vi "Main.vi"() -> ()   [LabVIEW 2017]
uses:
  <vilib>/addons/database/Connection.llb/Conn ObjectReference.ctl
  <vilib>/addons/database/Connection.llb/DB Tools Open Connec (Path).vi
  <vilib>/addons/database/Connection.llb/Conn Execute.vi
  <vilib>/addons/database/Recordset.llb/Rec Fetch Recordset Data (R).vi
  <vilib>/addons/database/Recordset.llb/Rec Destroy - Connection.vi
  <vilib>/addons/database/NI_Database_API.lvlib
panel:
  out "Current Time":string
  out "Current Date":string
  out "1D Array":string[](array[string])=["01:00 - 01:59", "02:00 - 02:59", "03:00 - 03:59", "04:00 - 04:59", "05:00 - 05:59", "06:00 - 06:59", "07:00 - 07:59", "08:00 - 08:59", "09:00 - 09:59", "10:00 - 10:59", "11:00 - 11:59", "12:00 - 12:59", "13:00 - 13:59", "14:00 - 14:59", "15:00 - 15:59", "16:00 - 16:59", "17:00 - 17:59", "18:00 - 18:59", "19:00 - 19:59", "20:00 - 20:59", "21:00 - 21:59", "22:00 - 22:59", "22:00 - 22:59", "00:00 - 01:59"]
  out "String Indicator 9":string="BREAKDOWN COUNT"
  out "String Indicator":string="PRODUCTION COUNT"
  out "String Indicator 8":string="REJECTION COUNT"
  out "Dlt Cnt":i32
  out "Table 2":string[][][](array[string])
  out "connection reference":T1
  out "String Indicator 1":string="RUNNING..."
  out "BDWn1":dbl
  out "Rej1":dbl
  out "Prod1":dbl
  out "Total Bdwn Time":timestamp format="%<%H:%M:%S>T"
  out "Hourly1":dbl[](array[numeric])
  out "BSWN3":dbl
  out "Rej3":dbl
  out "Prod 3":dbl
  out "Total Bdwn Time3":timestamp format="%<%H:%M:%S>T"
  out "String Indicator 3":string="RUNNING..."
  out "Hourly3":dbl[](array[numeric])
  out "BDWN2":dbl
  out "Rej2":dbl
  out "Prod 2":dbl
  out "Total Bdwn Time2":timestamp format="%<%H:%M:%S>T"
  out "String Indicator 2":string="RUNNING..."
  out "Hourly2":dbl[](array[numeric])
  out "BDWN6":dbl
  out "Rej6":dbl
  out "Prod6":dbl
  out "Total Bdwn Time4":timestamp format="%<%H:%M:%S>T"
  out "String Indicator 6":string="RUNNING..."
  out "Hourly6":dbl[](array[numeric])
  out "BDWN5":dbl
  out "Rej5":dbl
  out "Prod5":dbl
  out "Total Bdwn Time5":timestamp format="%<%H:%M:%S>T"
  out "String Indicator 5":string="RUNNING..."
  out "Hourly5":dbl[](array[numeric])
  out "BDWN4":dbl
  out "Rej4":dbl
  out "Prod4":dbl
  out "Total Bdwn Time6":timestamp format="%<%H:%M:%S>T"
  out "String Indicator4":string="RUNNING..."
  out "Hourly4":dbl[](array[numeric])
  out "Numeric Indicator 4":string=" BREAKDOWN TIME "
  out "Numeric Indicator 3":string="STATUS"
  in  "Cancel Button - Archive":bool
  # "Main Screen"
  # "Station_1"
  # "Station_2"
  # "Station_3"
  # "Station_4"
  # "Station_5"
  # "Station_6"
  # "Designed & Developed By: Infinity Automation Systems Pvt. Ltd."
  # "00.00.53\n00.00.25\n00.00.21\n00.00.15\n11\n7\n2\n8\n1.6\n49\n35\n32\n27"
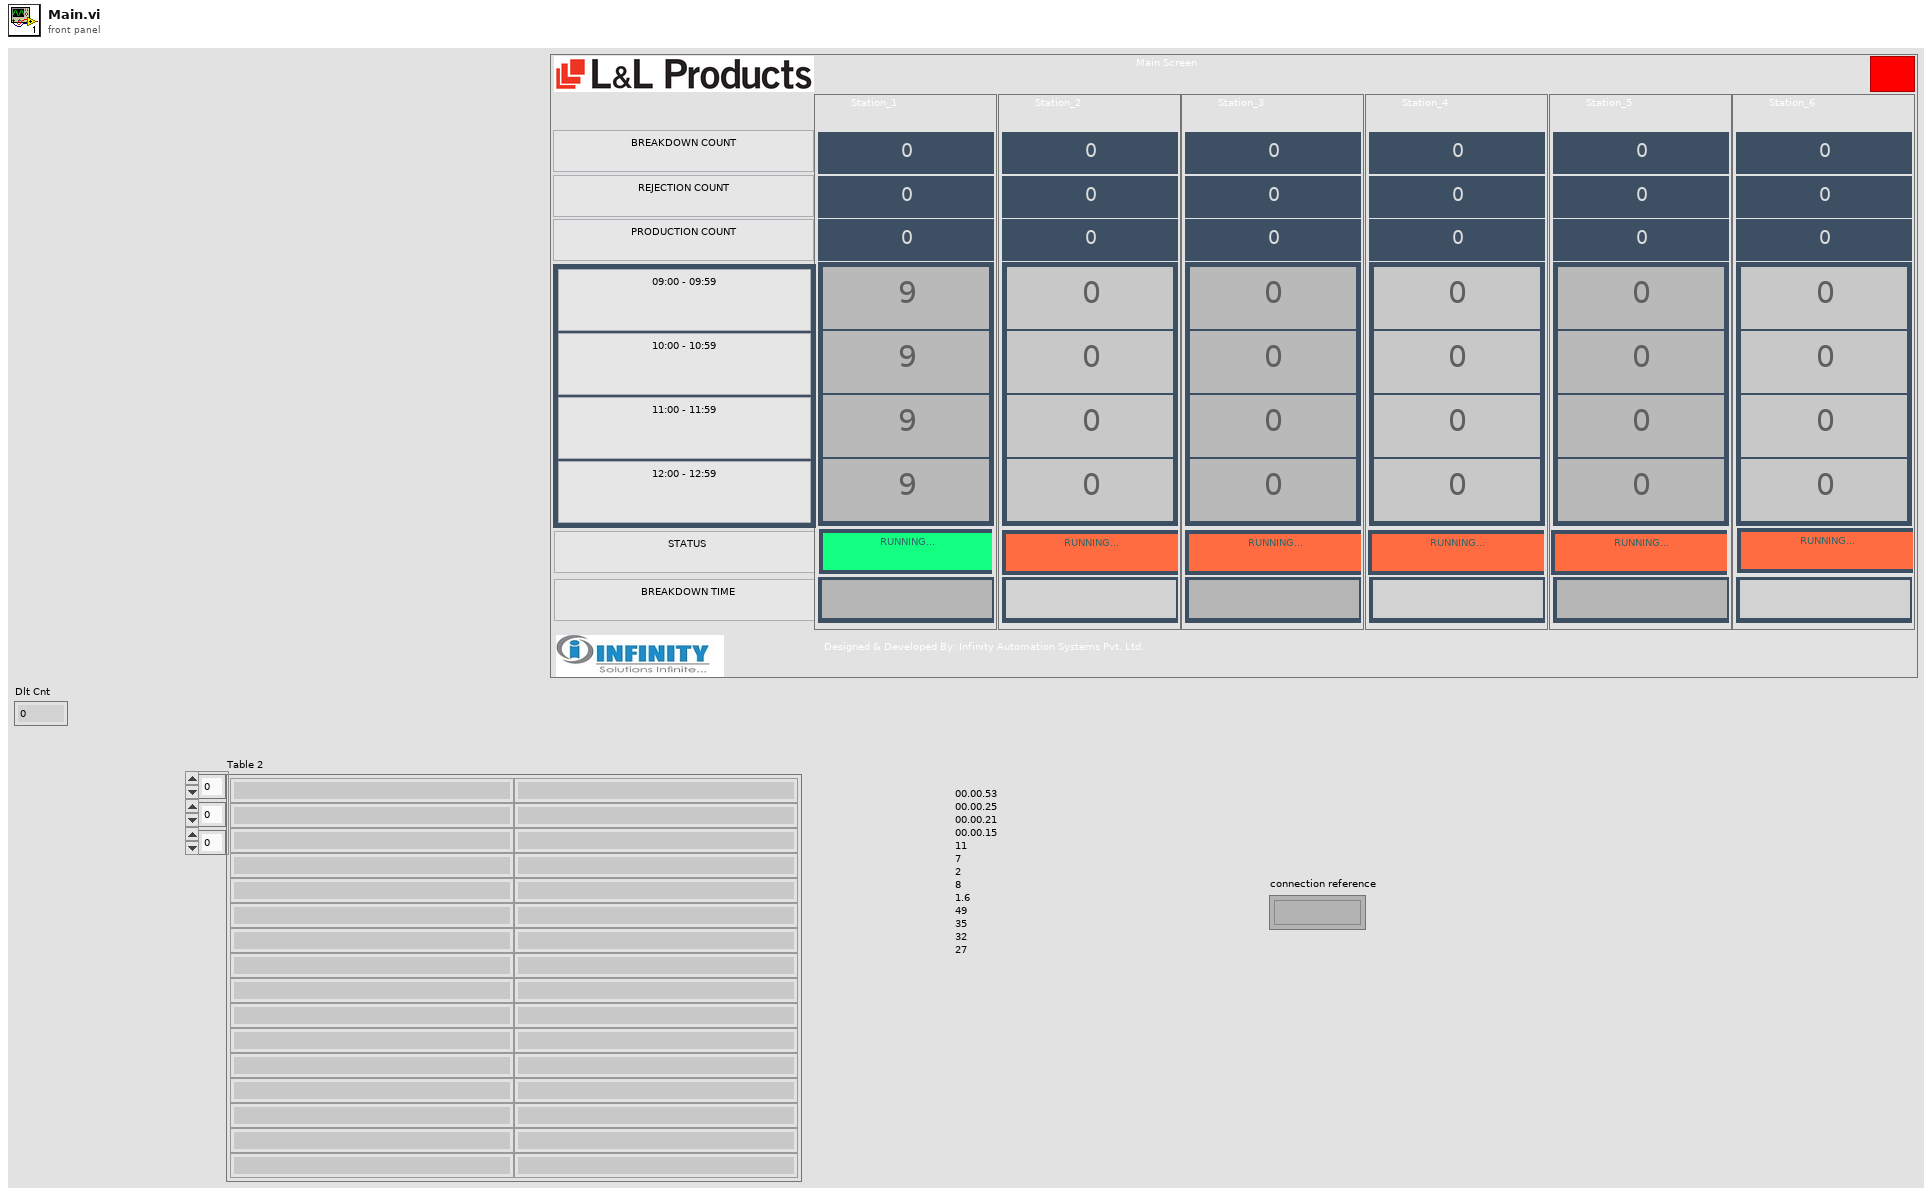
[diagram p1: front panel]
types:
  T1 = typedef "NI_Database_API.lvlib/Conn ObjectReference.ctl" = refnum<k1>
  T2 = typedef "NI_Database_API.lvlib/Rec ObjectReference.ctl" = refnum<k1>
  T3 = enum32{"invalid app kind", "Development System", "Run Time System", "Student Edition", "Embedded LabVIEW", "Evaluation", "Custom"}
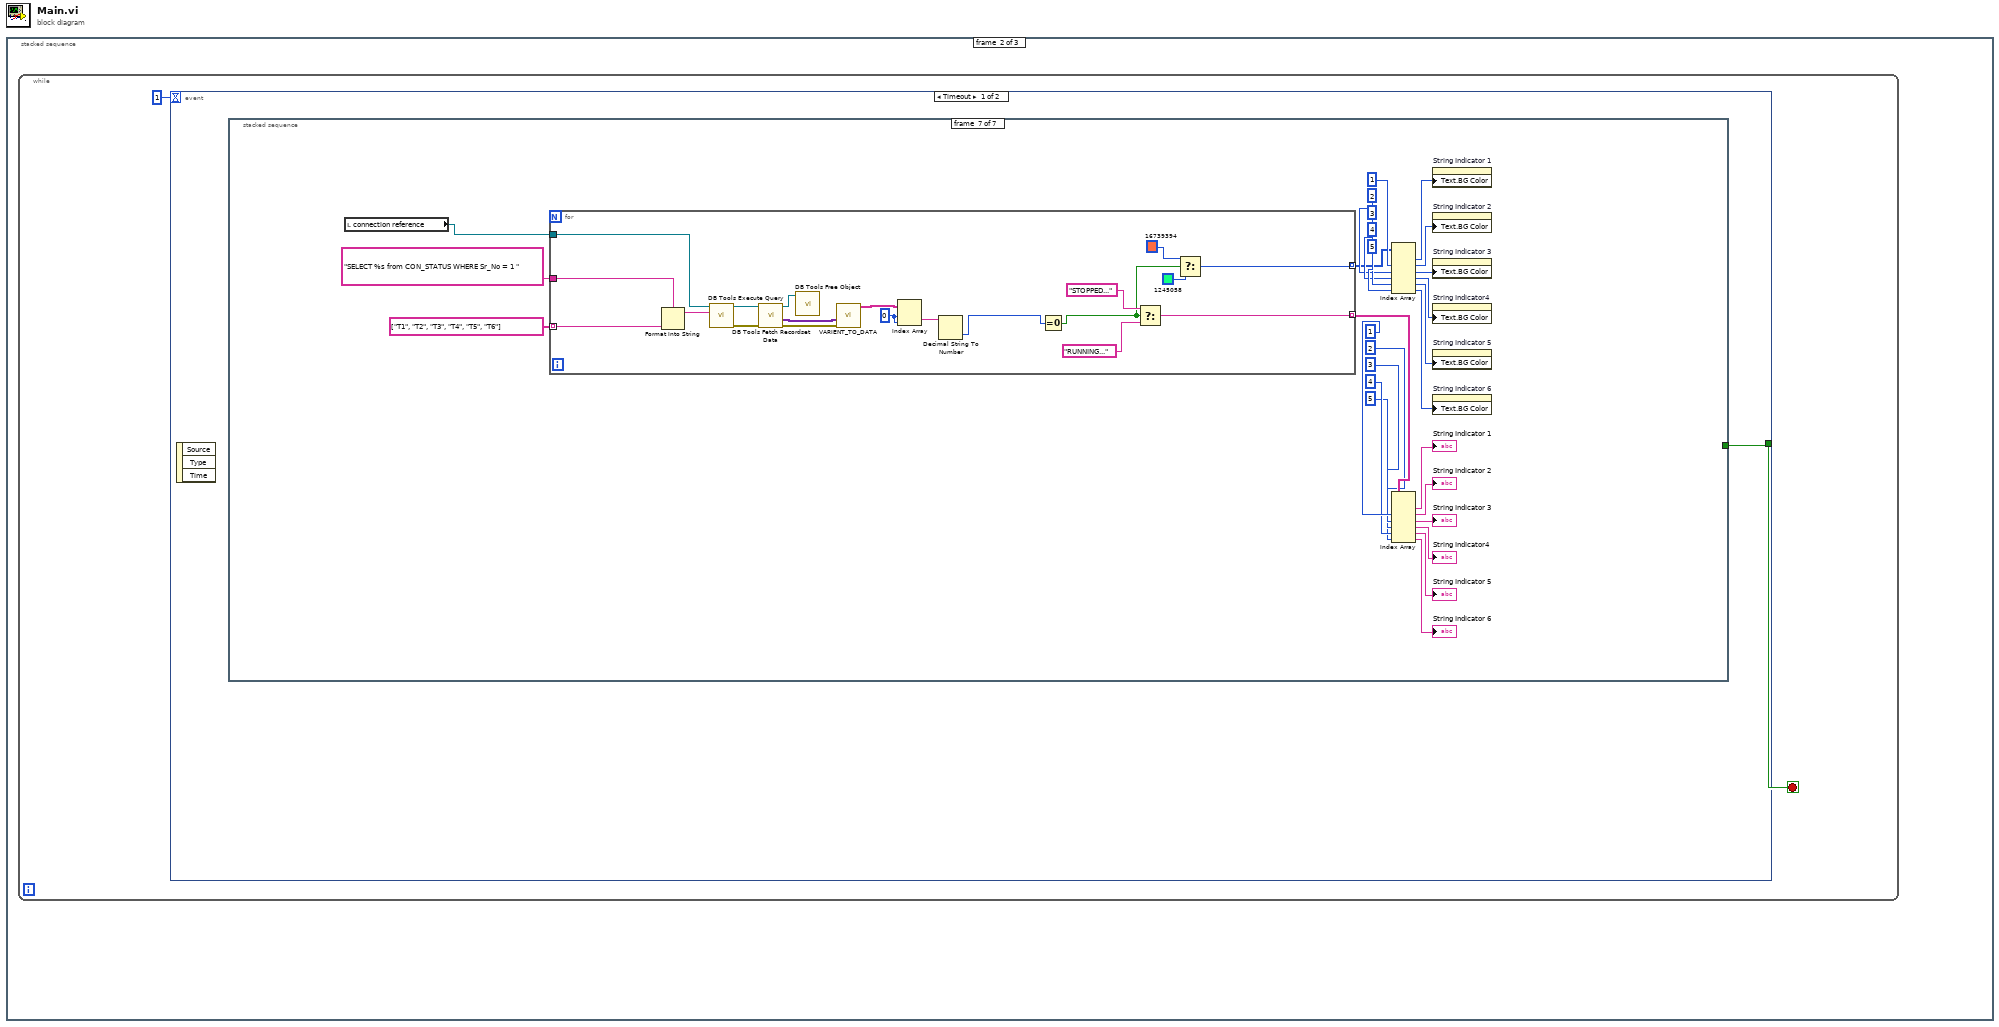
[diagram p0: block diagram]
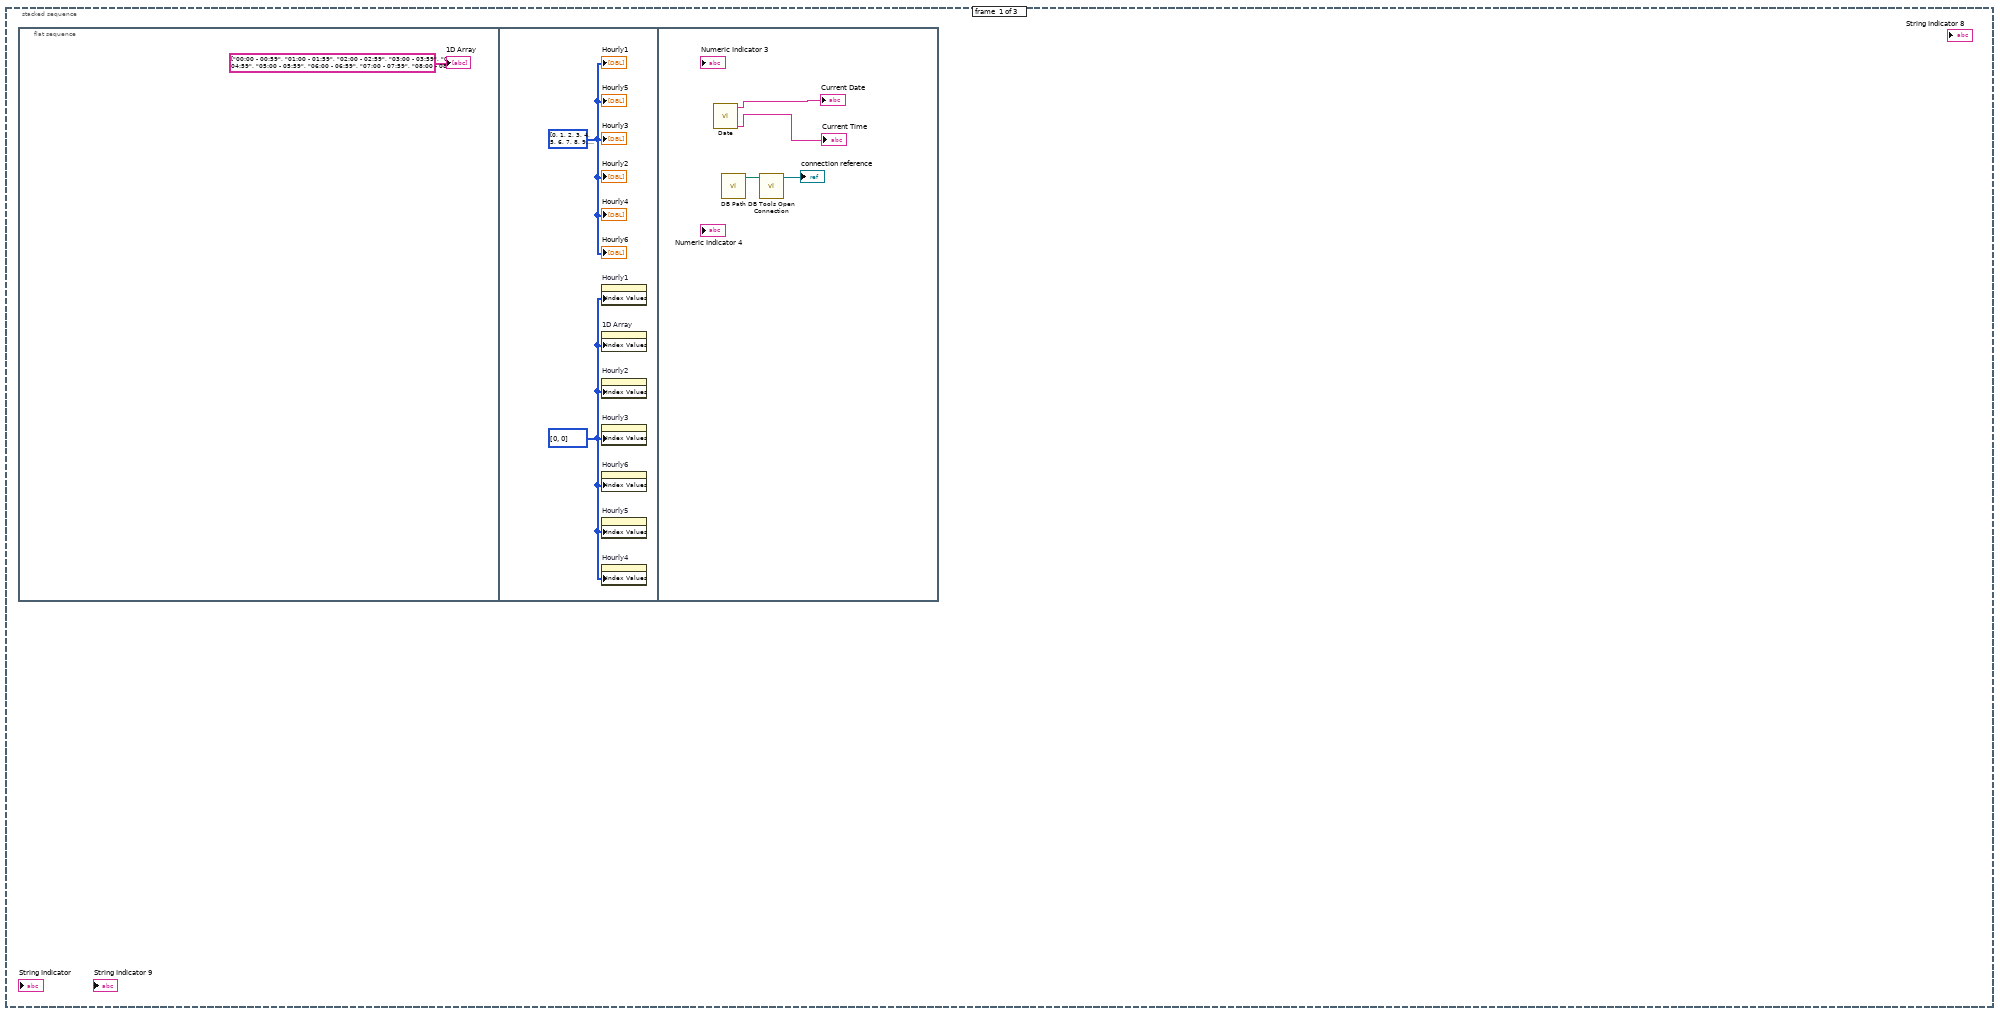
[diagram p2: hidden frame]
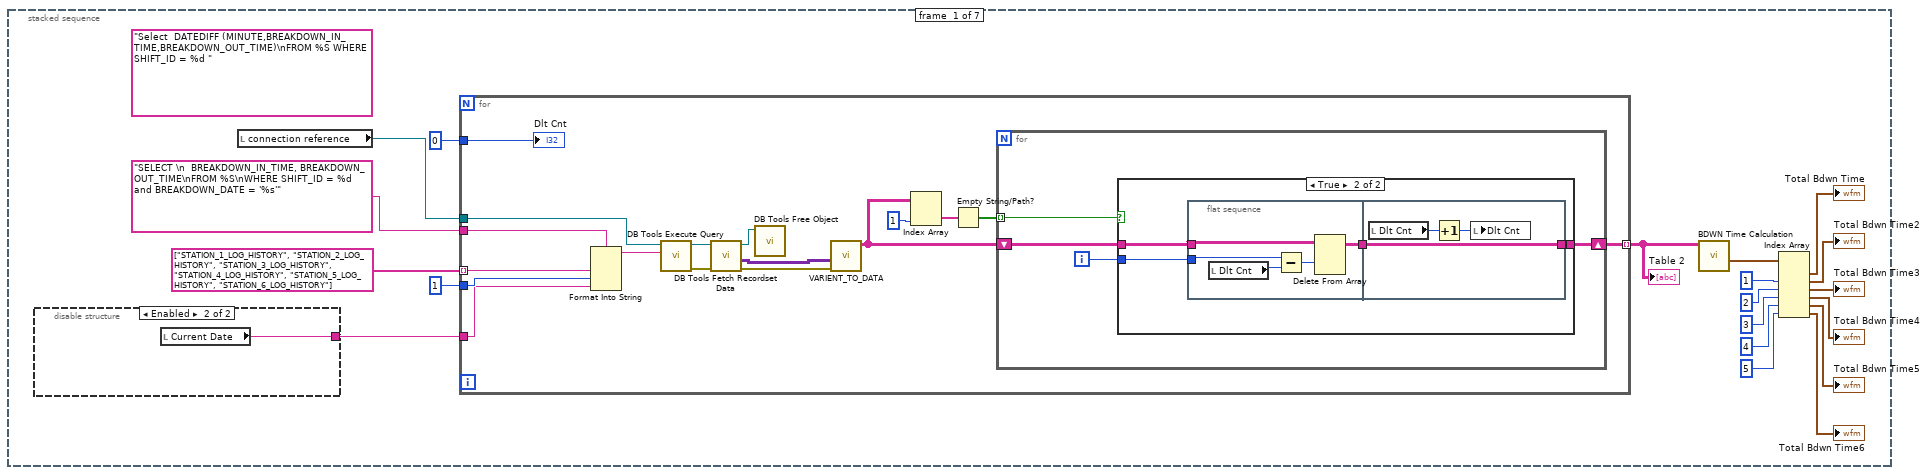
[diagram p3: hidden frame]
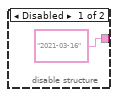
[diagram p4: hidden frame]
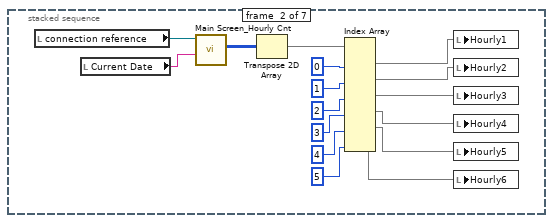
[diagram p6: hidden frame]
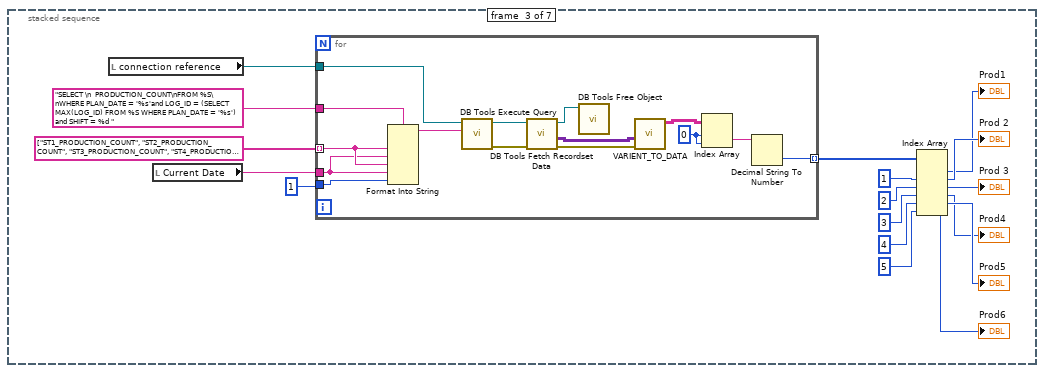
[diagram p7: hidden frame]
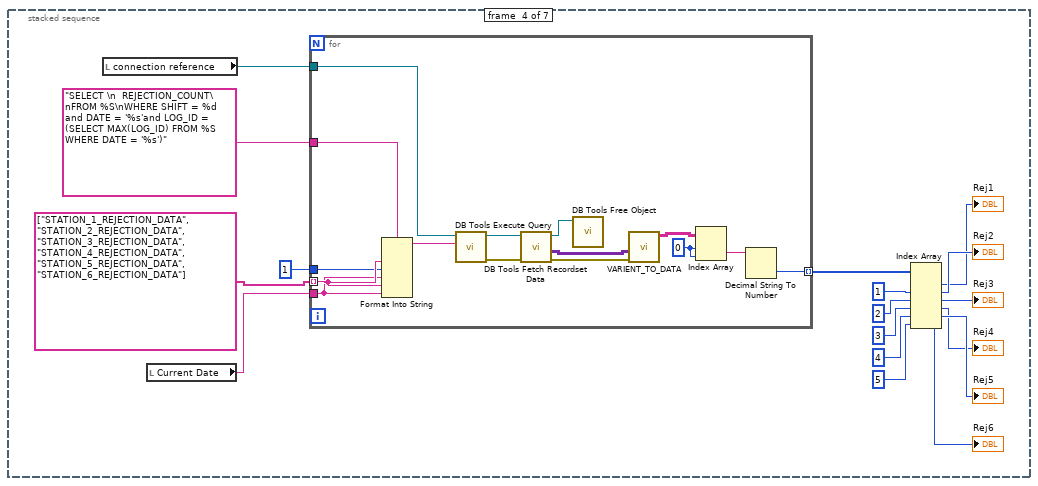
[diagram p8: hidden frame]
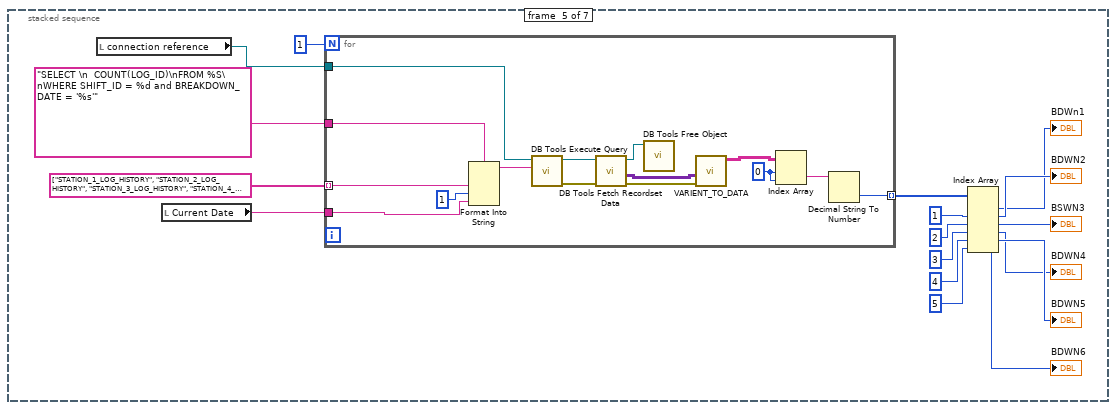
[diagram p9: hidden frame]
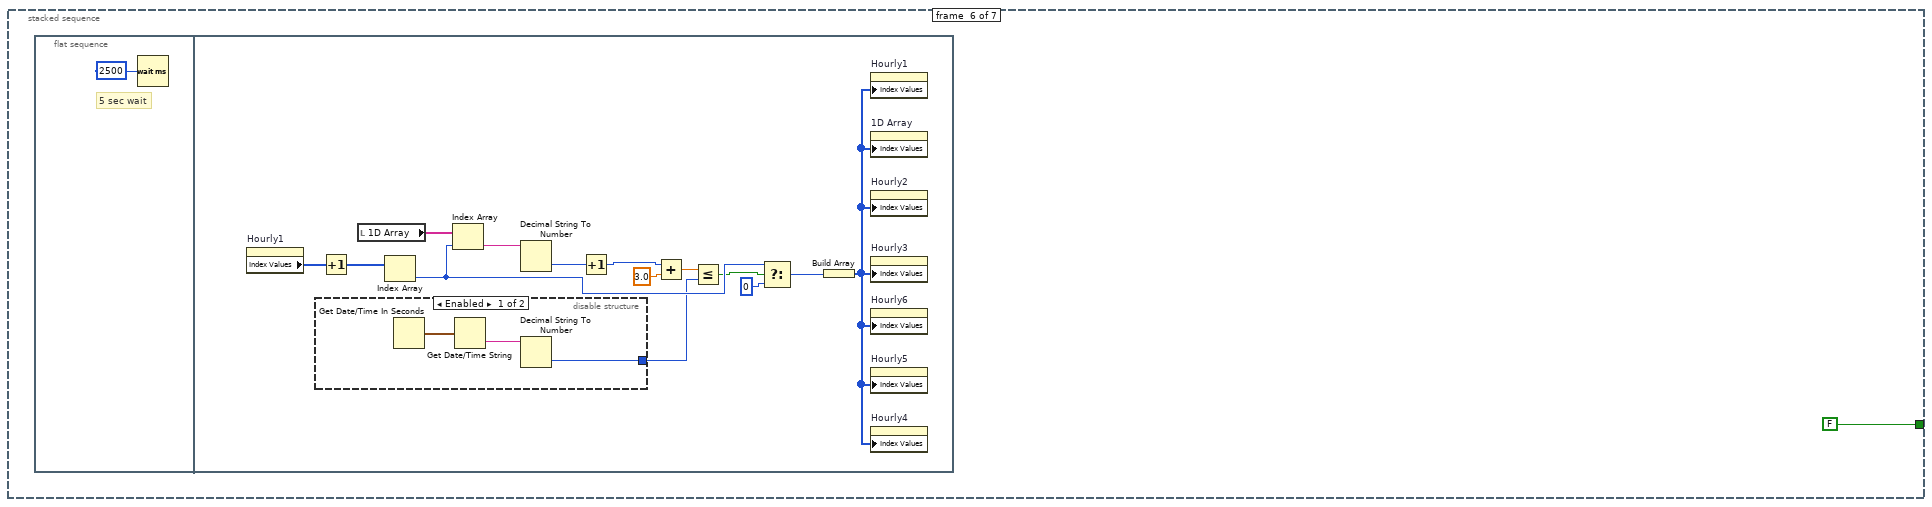
[diagram p10: hidden frame]
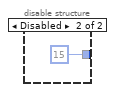
[diagram p11: hidden frame]
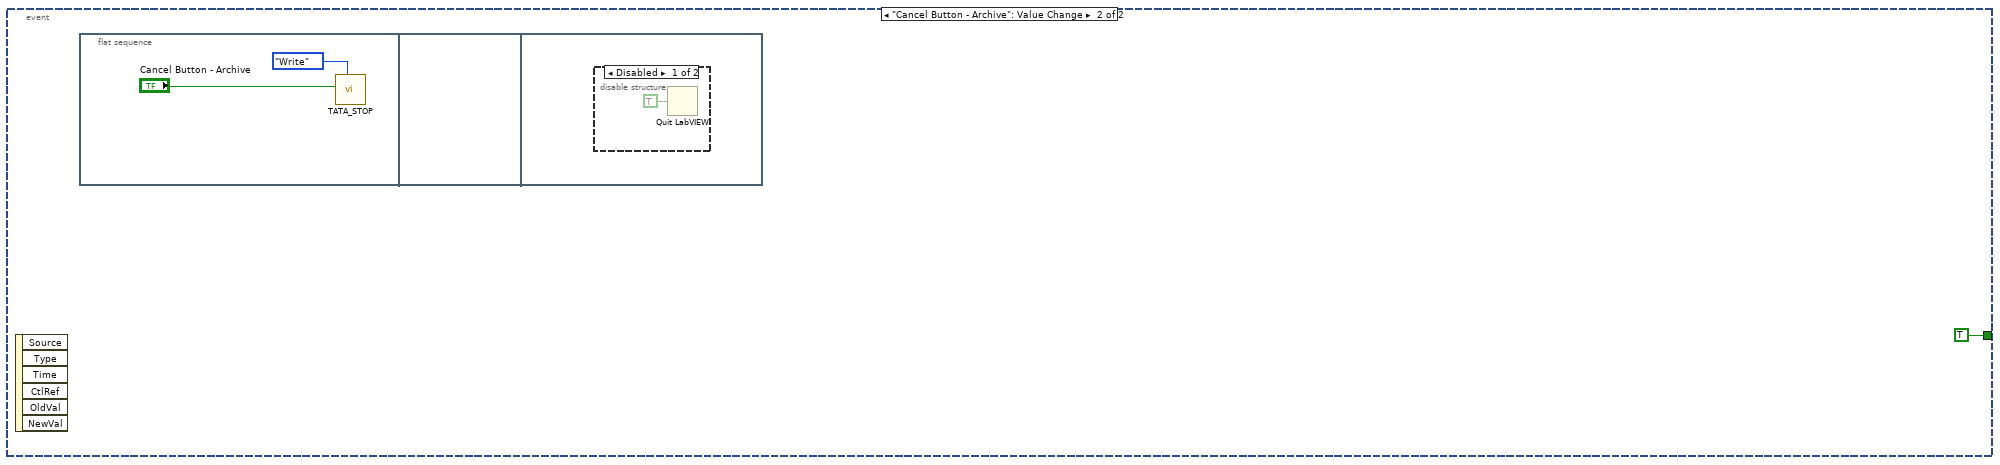
[diagram p12: hidden frame]
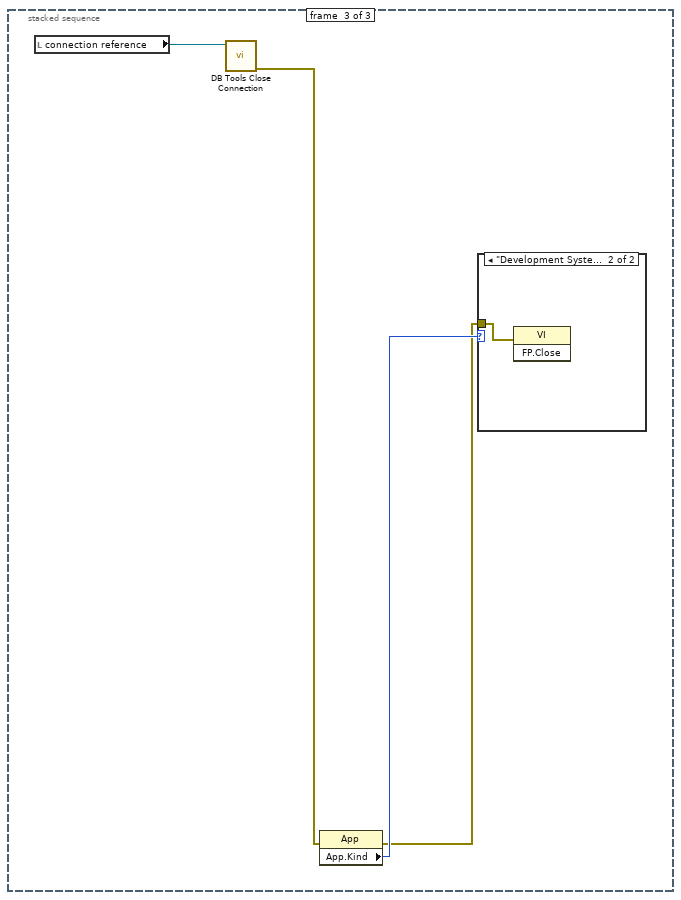
[diagram p14: hidden frame]
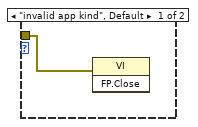
[diagram p15: hidden frame]
diagram:
  n1 = stacked-sequence {
    frame #0 {
      n2 = flat-sequence {
        frame #0 {
          "1D Array" <- string[] ["00:00 - 00:59", "01:00 - 01:59", "02:00 - 02:59", "03:00 - 03:59", "04:00 - 04:59", "05:00 - 05:59", "06:00 - 06:59", "07:00 - 07:59", "08:00 - 08:59", "09:00 - 09:59", "10:00 - 10:59", "11:00 - 11:59", "12:00 - 12:59", "13:00 - 13:59", "14:00 - 14:59", "15:00 - 15:59", "16:00 - 16:59", "17:00 - 17:59", "18:00 - 18:59", "19:00 - 19:59", "20:00 - 20:59", "21:00 - 21:59", "22:00 - 22:59", "23:00 - 23:59"] ("array w/ subset deleted")
        }
        frame #1 {
          w3 = u32[] [0, 1, 2, 3, 4, 5, 6, 7, 8, 9, 10] ("appended array")
          w2 = u32[] [0, 0] ("appended array")
          n3 = property on="Hourly1" class="Arr (strict)"("Index Values"=w2) -> ()  [unwired: 2 in, 2 out]
          n4 = property on="1D Array" class="Arr (strict)"("Index Values"=w2) -> ()  [unwired: 2 in, 2 out]
          n5 = property on="Hourly2" class="Arr (strict)"("Index Values"=w2) -> ()  [unwired: 2 in, 2 out]
          n6 = property on="Hourly3" class="Arr (strict)"("Index Values"=w2) -> ()  [unwired: 2 in, 2 out]
          n7 = property on="Hourly6" class="Arr (strict)"("Index Values"=w2) -> ()  [unwired: 2 in, 2 out]
          n8 = property on="Hourly5" class="Arr (strict)"("Index Values"=w2) -> ()  [unwired: 2 in, 2 out]
          n9 = property on="Hourly4" class="Arr (strict)"("Index Values"=w2) -> ()  [unwired: 2 in, 2 out]
          "Hourly1" <- w3
          "Hourly5" <- w3
          "Hourly3" <- w3
          "Hourly2" <- w3
          "Hourly4" <- w3
          "Hourly6" <- w3
        }
        frame #2 {
          n10 = call "Date.vi"() -> ("Current Time"=→"Current Time":string, "YYYYMMDD Date"=→"Current Date":string)  [unwired: 10 in]
          n11 = call "DB Path.vi"() -> ("DB Path"=w7:path)  [unwired: 10 in, 1 out]
          n12 = call-poly <vilib>:"DB Tools Open Connection.vi"("connection information"=w7) -> ("connection reference"=→"connection reference":T1)  [unwired: 7 in, 1 out]
        }
      }
    }
    frame #1 {
      n13 = while {
        stop <- w9 stop-if-true
        n14 = event shown="[0] Timeout" {
          selector: _ -> [_ _]
          dyn-events: _ -> [_ _]
          timeout: 1 -> [_ _]
          tunnel: [w10 TRUE] -> w9
          event Timeout {
            n15 = event-data() -> ()  [unwired: 1 in, 3 out]
            n16 = stacked-sequence {
              tunnel: [_ _ _ _ _ FALSE _] -> w10
              frame #0 {
                (unwired) "Select  DATEDIFF (MINUTE,BREAKDOWN_IN_TIME,BREAKDOWN_OUT_TIME)\nFROM %S WHERE SHIFT_ID = %d " ("SQL query")
                n17 = disable-structure shown="Enabled" {
                  disable-tunnel: ["2021-03-16" w31] -> w11
                  frame Disabled {
                  }
                  frame Enabled {
                    n18 = local read "Current Date"() -> (w31:string)
                  }
                }
                n19 = local read "connection reference"() -> (w28:T1)
                n20 = for {
                  tunnel: w28 -> [w48]
                  tunnel: "SELECT \n  BREAKDOWN_IN_TIME, BREAKDOWN_OUT_TIME\nFROM %S\nWHERE SHIFT_ID = %d and BREAKDOWN_DATE = '%s'" ("SQL query") -> [w44]
                  tunnel: string[] ["STATION_1_LOG_HISTORY", "STATION_2_LOG_HISTORY", "STATION_3_LOG_HISTORY", "STATION_4_LOG_HISTORY", "STATION_5_LOG_HISTORY", "STATION_6_LOG_HISTORY"] -> [w42] mode=indexing
                  tunnel: 1 ("input 2") -> [w41]
                  tunnel: 0 ("input 2") -> [w34]
                  tunnel: [w33] -> w25 mode=indexing
                  tunnel: w11 -> [w32]
                  n21 = Format Into String(format string=w44, w42, w41, w32) -> (resulting string=w43:string)  [unwired: 2 in, 1 out]
                  n22 = call-poly <vilib>:"DB Tools Execute Query.vi"("SQL query"=w43, "connection reference"=w48) -> ("error out"=w40:errorcluster, "recordset reference"=w47:T2)  [unwired: 6 in]
                  n23 = call-poly <vilib>:"DB Tools Fetch Recordset Data.vi"("error in (no error)"=w40, "recordset reference"=w47) -> ("error out"=w39:errorcluster, "recordset data"=w45:variant[][], "recordset reference out"=w46:T2)  [unwired: 3 in]
                  n24 = call-poly <vilib>:"DB Tools Free Object.vi"("recordset reference"=w46) -> ()  [unwired: 9 in, 2 out]
                  n25 = call "VARIENT_TO_DATA.vi"("data"=w45, "error in (no error)"=w39) -> ("Table"=w35:string[][])  [unwired: 7 in, 1 out]
                  n26 = Index Array(array=w35, index (col)=1 ("disabled index (col)")) -> (element=w37:string[])  [unwired: 1 in]
                  n27 = Empty String/Path?(string/path=w37) -> (empty?=w36:bool[])
                  n28 = for {
                    tunnel: w36 -> [w52] mode=indexing
                    shift-right: [w49] -> w33
                    shift-left: w35 -> [w51]
                    i -> [w50]
                    n29 = case shown="True" w52 {
                      tunnel: w51 -> [w53 w57]
                      tunnel: w50 -> [_ w56]
                      tunnel: [w53 w55] -> w49
                      frame False {
                      }
                      frame True {
                        n30 = flat-sequence {
                          tunnel: w57 -> [w62]
                          tunnel: w56 -> [w60]
                          tunnel: [w61] -> w54
                          tunnel: [w65] -> w55
                          tunnel: w54 -> [w65]
                          frame #0 {
                            n31 = local read "Dlt Cnt"() -> (w59:i32)
                            n32 = Subtract(x=w60, y=w59) -> (x-y=w58:i32)
                            n33 = Delete From Array(array=w62, index (row)=w58) -> (array with subset deleted=w61:string[][])  [unwired: 2 in, 1 out]
                          }
                          frame #1 {
                            n34 = local read "Dlt Cnt"() -> (w63:i32)
                            n35 = Increment(x=w63) -> (x+1=w64:i32)
                            n36 = local write "Dlt Cnt"(w64) -> ()
                          }
                        }
                      }
                    }
                  }
                  "Dlt Cnt" <- w34
                }
                "Table 2" <- w25
                n37 = call "BDWN Time Calculation.vi"("Input Table"=w25) -> ("All BDWN Time"=w24:timestamp[])  [unwired: 8 in, 1 out]
                n38 = Index Array(array=w24, index #2=1 ("index"), index #3=2 ("index"), index #4=3 ("index"), index #5=4 ("index"), index #6=5 ("index")) -> (element #1=→"Total Bdwn Time":timestamp, element #2=→"Total Bdwn Time2":timestamp, element #3=→"Total Bdwn Time3":timestamp, element #4=→"Total Bdwn Time4":timestamp, element #5=→"Total Bdwn Time5":timestamp, element #6=→"Total Bdwn Time6":timestamp)  [unwired: 1 in]
              }
              frame #1 {
                n39 = local read "connection reference"() -> (w73:T1)
                n40 = local read "Current Date"() -> (w66:string)
                n41 = call "Main Screen_Hourly Cnt.vi"("Current Date"=w66, "connection reference 2"=w73) -> ("Station Wise Max"=w74:i32[][])  [unwired: 9 in]
                n42 = Transpose 2D Array(2D array=w74) -> (transposed array=w75:i32[][])
                n43 = Index Array(array=w75, index (col) #1=0 ("disabled index (col)"), index (col) #2=1 ("index (col)"), index (col) #3=2 ("index (col)"), index (col) #4=3 ("index (col)"), index (col) #5=4 ("index (col)"), index (col) #6=5 ("index (col)")) -> (element #1=w76:i32[], element #2=w77:i32[], element #3=w78:i32[], element #4=w79:i32[], element #5=w80:i32[], element #6=w81:i32[])  [unwired: 6 in]
                n44 = local write "Hourly1"(w76) -> ()
                n45 = local write "Hourly2"(w77) -> ()
                n46 = local write "Hourly3"(w78) -> ()
                n47 = local write "Hourly4"(w79) -> ()
                n48 = local write "Hourly5"(w80) -> ()
                n49 = local write "Hourly6"(w81) -> ()
              }
              frame #2 {
                n50 = local read "connection reference"() -> (w98:T1)
                n51 = local read "Current Date"() -> (w82:string)
                n52 = for {
                  tunnel: w98 -> [w113]
                  tunnel: "SELECT \n  PRODUCTION_COUNT\nFROM %S\nWHERE PLAN_DATE = '%s'and LOG_ID = (SELECT MAX(LOG_ID) FROM %S WHERE PLAN_DATE = '%s') and SHIFT = %d " ("SQL query") -> [w109]
                  tunnel: string[] ["ST1_PRODUCTION_COUNT", "ST2_PRODUCTION_COUNT", "ST3_PRODUCTION_COUNT", "ST4_PRODUCTION_COUNT", "ST5_PRODUCTION_COUNT", "ST6_PRODUCTION_COUNT"] -> [w101] mode=indexing
                  tunnel: [w104] -> w91 mode=indexing
                  tunnel: w82 -> [w100]
                  tunnel: 1 ("index") -> [w99]
                  w106 = 0 ("index (row)")
                  n53 = Format Into String(format string=w109, w101, w100, w101, w100, w99) -> (resulting string=w108:string)  [unwired: 2 in, 1 out]
                  n54 = call-poly <vilib>:"DB Tools Execute Query.vi"("SQL query"=w108, "connection reference"=w113) -> ("error out"=w103:errorcluster, "recordset reference"=w112:T2)  [unwired: 6 in]
                  n55 = call-poly <vilib>:"DB Tools Fetch Recordset Data.vi"("error in (no error)"=w103, "recordset reference"=w112) -> ("error out"=w102:errorcluster, "recordset data"=w110:variant[][], "recordset reference out"=w111:T2)  [unwired: 3 in]
                  n56 = call-poly <vilib>:"DB Tools Free Object.vi"("recordset reference"=w111) -> ()  [unwired: 9 in, 2 out]
                  n57 = call "VARIENT_TO_DATA.vi"("data"=w110, "error in (no error)"=w102) -> ("Table"=w107:string[][])  [unwired: 7 in, 1 out]
                  n58 = Index Array(array=w107, index (row)=w106, index (col)=w106) -> (element=w105:string)
                  n59 = Decimal String To Number(string=w105) -> (number=w104:i32)  [unwired: 2 in, 1 out]
                }
                n60 = Index Array(array=w91, index #2=1 ("index"), index #3=2 ("index"), index #4=3 ("index"), index #5=4 ("index"), index #6=5 ("index")) -> (element #1=→"Prod1":i32, element #2=→"Prod 2":i32, element #3=→"Prod 3":i32, element #4=→"Prod4":i32, element #5=→"Prod5":i32, element #6=→"Prod6":i32)  [unwired: 1 in]
              }
              frame #3 {
                n61 = local read "connection reference"() -> (w130:T1)
                n62 = local read "Current Date"() -> (w114:string)
                n63 = for {
                  tunnel: w130 -> [w145]
                  tunnel: "SELECT \n  REJECTION_COUNT\nFROM %S\nWHERE SHIFT = %d and DATE = '%s'and LOG_ID = (SELECT MAX(LOG_ID) FROM %S WHERE DATE = '%s')" ("SQL query") -> [w141]
                  tunnel: string[] ["STATION_1_REJECTION_DATA", "STATION_2_REJECTION_DATA", "STATION_3_REJECTION_DATA", "STATION_4_REJECTION_DATA", "STATION_5_REJECTION_DATA", "STATION_6_REJECTION_DATA"] -> [w133] mode=indexing
                  tunnel: [w136] -> w123 mode=indexing
                  tunnel: w114 -> [w131]
                  tunnel: 1 ("index") -> [w132]
                  w138 = 0 ("index (row)")
                  n64 = Format Into String(format string=w141, w133, w132, w131, w133, w131) -> (resulting string=w140:string)  [unwired: 2 in, 1 out]
                  n65 = call-poly <vilib>:"DB Tools Execute Query.vi"("SQL query"=w140, "connection reference"=w145) -> ("error out"=w135:errorcluster, "recordset reference"=w144:T2)  [unwired: 6 in]
                  n66 = call-poly <vilib>:"DB Tools Fetch Recordset Data.vi"("error in (no error)"=w135, "recordset reference"=w144) -> ("error out"=w134:errorcluster, "recordset data"=w142:variant[][], "recordset reference out"=w143:T2)  [unwired: 3 in]
                  n67 = call-poly <vilib>:"DB Tools Free Object.vi"("recordset reference"=w143) -> ()  [unwired: 9 in, 2 out]
                  n68 = call "VARIENT_TO_DATA.vi"("data"=w142, "error in (no error)"=w134) -> ("Table"=w139:string[][])  [unwired: 7 in, 1 out]
                  n69 = Index Array(array=w139, index (row)=w138, index (col)=w138) -> (element=w137:string)
                  n70 = Decimal String To Number(string=w137) -> (number=w136:i32)  [unwired: 2 in, 1 out]
                }
                n71 = Index Array(array=w123, index #2=1 ("index"), index #3=2 ("index"), index #4=3 ("index"), index #5=4 ("index"), index #6=5 ("index")) -> (element #1=→"Rej1":i32, element #2=→"Rej2":i32, element #3=→"Rej3":i32, element #4=→"Rej4":i32, element #5=→"Rej5":i32, element #6=→"Rej6":i32)  [unwired: 1 in]
              }
              frame #4 {
                n72 = local read "connection reference"() -> (w156:T1)
                n73 = local read "Current Date"() -> (w146:string)
                n74 = for {
                  N: 1 -> [_]
                  tunnel: w156 -> [w177]
                  tunnel: "SELECT \n  COUNT(LOG_ID)\nFROM %S\nWHERE SHIFT_ID = %d and BREAKDOWN_DATE = '%s'" ("SQL query") -> [w173]
                  tunnel: string[] ["STATION_1_LOG_HISTORY", "STATION_2_LOG_HISTORY", "STATION_3_LOG_HISTORY", "STATION_4_LOG_HISTORY", "STATION_5_LOG_HISTORY", "STATION_6_LOG_HISTORY"] -> [w165] mode=indexing
                  tunnel: [w168] -> w155 mode=indexing
                  tunnel: w146 -> [w164]
                  w170 = 0 ("index (row)")
                  n75 = Format Into String(format string=w173, w165, 1 ("input 2"), w164) -> (resulting string=w172:string)  [unwired: 2 in, 1 out]
                  n76 = call-poly <vilib>:"DB Tools Execute Query.vi"("SQL query"=w172, "connection reference"=w177) -> ("error out"=w167:errorcluster, "recordset reference"=w176:T2)  [unwired: 6 in]
                  n77 = call-poly <vilib>:"DB Tools Fetch Recordset Data.vi"("error in (no error)"=w167, "recordset reference"=w176) -> ("error out"=w166:errorcluster, "recordset data"=w174:variant[][], "recordset reference out"=w175:T2)  [unwired: 3 in]
                  n78 = call-poly <vilib>:"DB Tools Free Object.vi"("recordset reference"=w175) -> ()  [unwired: 9 in, 2 out]
                  n79 = call "VARIENT_TO_DATA.vi"("data"=w174, "error in (no error)"=w166) -> ("Table"=w171:string[][])  [unwired: 7 in, 1 out]
                  n80 = Index Array(array=w171, index (row)=w170, index (col)=w170) -> (element=w169:string)
                  n81 = Decimal String To Number(string=w169) -> (number=w168:i32)  [unwired: 2 in, 1 out]
                }
                n82 = Index Array(array=w155, index #2=1 ("index"), index #3=2 ("index"), index #4=3 ("index"), index #5=4 ("index"), index #6=5 ("index")) -> (element #1=→"BDWn1":i32, element #2=→"BDWN2":i32, element #3=→"BSWN3":i32, element #4=→"BDWN4":i32, element #5=→"BDWN5":i32, element #6=→"BDWN6":i32)  [unwired: 1 in]
              }
              frame #5 {
                n83 = flat-sequence {
                  frame #0 {
                    # "5 sec wait"
                    n84 = Wait (ms)(milliseconds to wait=u32 2500) -> ()  [unwired: 1 out]
                  }
                  frame #1 {
                    n85 = property on="Hourly1" class="Arr (strict)"() -> ("Index Values"=w193:u32[])  [unwired: 2 in, 2 out]
                    n86 = disable-structure shown="Enabled" {
                      disable-tunnel: [w194 15] -> w184
                      frame Enabled {
                        n87 = Get Date/Time In Seconds() -> (seconds since 1Jan1904=w196:timestamp)
                        n88 = Get Date/Time String(seconds (now)=w196) -> (time string=w195:string)  [unwired: 2 in, 1 out]
                        n89 = Decimal String To Number(string=w195) -> (number=w194:i32)  [unwired: 2 in, 1 out]
                      }
                      frame Disabled {
                      }
                    }
                    n90 = Increment(x=w193) -> (x+1=w192:u32[])
                    n91 = local read "1D Array"() -> (w189:string[])
                    n92 = Index Array(array=w192) -> (element=w188:u32)  [unwired: 1 in]
                    n93 = Index Array(array=w189, index=w188) -> (element=w187:string)
                    n94 = Decimal String To Number(string=w187) -> (number=w186:i32)  [unwired: 2 in, 1 out]
                    n95 = Increment(x=w186) -> (x+1=w182:i32)
                    n96 = Add(x=w182, y=3.0) -> (x+y=w181:dbl)
                    n97 = Less Or Equal?(x=w181, y=w184) -> (x <= y?=w185:bool)
                    n98 = Select(t=w188, s=w185, f=u32 0) -> (s? t:f=w190:u32)
                    n99 = Build Array(w190) -> (w180:u32[])
                    n100 = property on="Hourly1" class="Arr (strict)"("Index Values"=w180) -> ()  [unwired: 2 in, 2 out]
                    n101 = property on="1D Array" class="Arr (strict)"("Index Values"=w180) -> ()  [unwired: 2 in, 2 out]
                    n102 = property on="Hourly2" class="Arr (strict)"("Index Values"=w180) -> ()  [unwired: 2 in, 2 out]
                    n103 = property on="Hourly3" class="Arr (strict)"("Index Values"=w180) -> ()  [unwired: 2 in, 2 out]
                    n104 = property on="Hourly6" class="Arr (strict)"("Index Values"=w180) -> ()  [unwired: 2 in, 2 out]
                    n105 = property on="Hourly5" class="Arr (strict)"("Index Values"=w180) -> ()  [unwired: 2 in, 2 out]
                    n106 = property on="Hourly4" class="Arr (strict)"("Index Values"=w180) -> ()  [unwired: 2 in, 2 out]
                  }
                }
              }
              frame #6 {
                n107 = local read "connection reference"() -> (w224:T1)
                n108 = for {
                  tunnel: w224 -> [w244]
                  tunnel: "SELECT %s from CON_STATUS WHERE Sr_No = 1 " ("SQL query") -> [w240]
                  tunnel: string[] ["T1", "T2", "T3", "T4", "T5", "T6"] -> [w233] mode=indexing
                  tunnel: [w229] -> w221 mode=indexing
                  tunnel: [w225] -> w204 mode=indexing
                  w237 = 0 ("index (row)")
                  n109 = Format Into String(format string=w240, w233) -> (resulting string=w239:string)  [unwired: 2 in, 1 out]
                  n110 = call-poly <vilib>:"DB Tools Execute Query.vi"("SQL query"=w239, "connection reference"=w244) -> ("error out"=w235:errorcluster, "recordset reference"=w243:T2)  [unwired: 6 in]
                  n111 = call-poly <vilib>:"DB Tools Fetch Recordset Data.vi"("error in (no error)"=w235, "recordset reference"=w243) -> ("error out"=w234:errorcluster, "recordset data"=w241:variant[][], "recordset reference out"=w242:T2)  [unwired: 3 in]
                  n112 = call-poly <vilib>:"DB Tools Free Object.vi"("recordset reference"=w242) -> ()  [unwired: 9 in, 2 out]
                  n113 = call "VARIENT_TO_DATA.vi"("data"=w241, "error in (no error)"=w234) -> ("Table"=w238:string[][])  [unwired: 7 in, 1 out]
                  n114 = Index Array(array=w238, index (row)=w237, index (col)=w237) -> (element=w236:string)
                  n115 = Decimal String To Number(string=w236) -> (number=w232:i32)  [unwired: 2 in, 1 out]
                  n116 = Equal To 0?(x=w232) -> (x = 0?=w228:bool)
                  n117 = Select(t="STOPPED..." ("String Indicator 1"), s=w228, f="RUNNING..." ("String Indicator 1")) -> (s? t:f=w229:string)
                  n118 = Select(t=u32 16739394, s=w228, f=u32 1245058) -> (s? t:f=w225:u32)
                }
                n119 = Index Array(array=w204, index #2=1 ("index"), index #3=2 ("index"), index #4=3 ("index"), index #5=4 ("index"), index #6=5 ("index")) -> (element #1=w203:u32, element #2=w202:u32, element #3=w201:u32, element #4=w200:u32, element #5=w199:u32, element #6=w198:u32)  [unwired: 1 in]
                n120 = Index Array(array=w221, index #2=1 ("index"), index #3=2 ("index"), index #4=3 ("index"), index #5=4 ("index"), index #6=5 ("index")) -> (element #1=→"String Indicator 1":string, element #2=→"String Indicator 2":string, element #3=→"String Indicator 3":string, element #4=→"String Indicator4":string, element #5=→"String Indicator 5":string, element #6=→"String Indicator 6":string)  [unwired: 1 in]
                n121 = property on="String Indicator 1" class="Str"("Text.BG Color"=w203) -> ()  [unwired: 2 in, 2 out]
                n122 = property on="String Indicator 2" class="Str"("Text.BG Color"=w202) -> ()  [unwired: 2 in, 2 out]
                n123 = property on="String Indicator 3" class="Str"("Text.BG Color"=w201) -> ()  [unwired: 2 in, 2 out]
                n124 = property on="String Indicator4" class="Str"("Text.BG Color"=w200) -> ()  [unwired: 2 in, 2 out]
                n125 = property on="String Indicator 5" class="Str"("Text.BG Color"=w199) -> ()  [unwired: 2 in, 2 out]
                n126 = property on="String Indicator 6" class="Str"("Text.BG Color"=w198) -> ()  [unwired: 2 in, 2 out]
              }
            }
          }
          event "Cancel Button - Archive": Value Change {
            n127 = event-data() -> ()  [unwired: 1 in, 6 out]
            n128 = flat-sequence {
              frame #0 {
                n129 = call "TATA_STOP.vi"("Enum"=enum16{"Read", "Write"}."Write", "Boolean"="Cancel Button - Archive") -> ()  [unwired: 8 in, 2 out]
              }
              frame #1 {
              }
              frame #2 {
                n130 = disable-structure shown="Disabled" {
                  frame Disabled {
                    n131 = Quit LabVIEW(quit? (T)=TRUE) -> ()
                  }
                  frame Enabled {
                  }
                }
              }
            }
          }
        }
      }
    }
    frame #2 {
      n132 = local read "connection reference"() -> (w252:T1)
      n133 = call <vilib>:"DB Tools Close Connection.vi"("connection reference"=w252) -> ("error out"=w250:errorcluster)  [unwired: 6 in]
      n134 = property class="App"(error in=w250) -> (error out=w249:errorcluster, "App.Kind"=w251:T3)  [unwired: 1 in, 1 out]
      n135 = case shown="\"Development System\"" w251 {
        tunnel: w249 -> [w253 w254]
        frame "invalid app kind", Default {
          n136 = invoke class="VI" method="FP.Close"(error in=w253) -> ()  [unwired: 2 in, 3 out]
        }
        frame "Development System" {
          n137 = invoke class="VI" method="FP.Close"(error in=w254) -> ()  [unwired: 2 in, 3 out]
        }
      }
    }
  }
